vi "Teleop.vi"(10 "Match Info":T1={"Autonomous Elapsed Seconds"=0.0, "TeleOp Elapsed Seconds"=0.0, "Disabled Elapsed Seconds"=0.0, "Visited Autonomous"=FALSE, "Visited TeleOp"=FALSE, "Visited Disabled"=FALSE, "Autonomous Settings"={"Autonomous Style"=enum."Independent", "VI Refnum"=refnum}}, 11 "Call Context":T2) -> ()   [LabVIEW 2015]
doc: "This VI is called for each TeleOp packet received from the DS where the robot is not disabled. It is often used to read from the joysticks and update I/O or to update setpoints for timed control loops. It should complete and return within 20 milliseconds or it may miss DS packets."
uses:
  <vilib>/Rock Robotics/WPI/DriverStation/WPI_DriverStationDerivedRobotMode.ctl
  <vilib>/Rock Robotics/WPI/DriverStation/WPI_DriverStationMatch Info.ctl
  <vilib>/Rock Robotics/WPI/Solenoid/WPI_SolenoidValue.ctl
  <vilib>/Rock Robotics/WPI/Utilities/WPI_GetSetVariantRefNum.vi
  <vilib>/Rock Robotics/Network Tables/NT Write Boolean Array.vi
  <vilib>/Rock Robotics/Network Tables/NT Write Numeric Array.vi
  <vilib>/Rock Robotics/Network Tables/NT Read Boolean.vi
  <vilib>/Rock Robotics/Network Tables/NT Read Number.vi
  Robot Global Data.vi
  <vilib>/Rock Robotics/WPI/Solenoid/WPI_SolenoidSetEnum.vi
panel:
  in  "Delay (ms)":u32=5000
  in  "ArmFactor":dbl=1.0
  in  "y":dbl
  in  "WinchFactor":dbl=-1.0 format="%#_13g"
  in  "SquareInput?":bool
  in  "Rumble":sgl
  out "Sample Slider 0":dbl(slide) scale=0.0..5.0
  out "Sample Boolean 1":bool
  out "Sample Boolean 0":bool
  # "h"
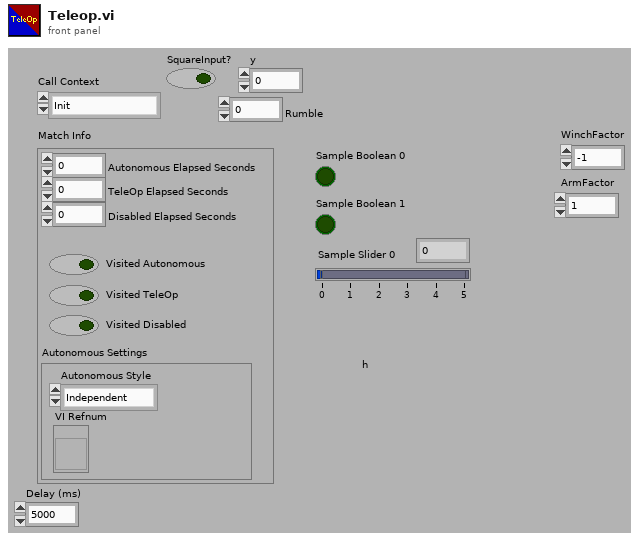
[diagram p1: front panel]
types:
  T1 = typedef "WPI_DriverStationMatch Info.ctl" = cluster{"Autonomous Elapsed Seconds":dbl, "TeleOp Elapsed Seconds":dbl, "Disabled Elapsed Seconds":dbl, "Visited Autonomous":bool, "Visited TeleOp":bool, "Visited Disabled":bool, "Autonomous Settings":cluster{"Autonomous Style":enum16{"Iterative", "Independent"}, "VI Refnum":refnum<vi>}}
  T2 = typedef "WPI_DriverStationDerivedRobotMode.ctl" = enum16{"Init", "Execute", "Stop"}
  T3 = cluster{"Distance (ft)":dbl, "Center":cluster{dbl, dbl}, "Normalized Rect":cluster{"Numeric":dbl, "Numeric 2":dbl, "Numeric 3":dbl, "Numeric 5":dbl}}[]
  T4 = cluster{"Detected Targets[0]":cluster{"Distance (ft)":dbl, "Center":cluster{dbl, dbl}, "Normalized Rect":cluster{"Numeric":dbl, "Numeric 2":dbl, "Numeric 3":dbl, "Numeric 5":dbl}}, "Detected Targets[1]":cluster{"Distance (ft)":dbl, "Center":cluster{dbl, dbl}, "Normalized Rect":cluster{"Numeric":dbl, "Numeric 2":dbl, "Numeric 3":dbl, "Numeric 5":dbl}}, "Detected Targets[2]":cluster{"Distance (ft)":dbl, "Center":cluster{dbl, dbl}, "Normalized Rect":cluster{"Numeric":dbl, "Numeric 2":dbl, "Numeric 3":dbl, "Numeric 5":dbl}}, "Detected Targets[3]":cluster{"Distance (ft)":dbl, "Center":cluster{dbl, dbl}, "Normalized Rect":cluster{"Numeric":dbl, "Numeric 2":dbl, "Numeric 3":dbl, "Numeric 5":dbl}}, "Detected Targets[4]":cluster{"Distance (ft)":dbl, "Center":cluster{dbl, dbl}, "Normalized Rect":cluster{"Numeric":dbl, "Numeric 2":dbl, "Numeric 3":dbl, "Numeric 5":dbl}}, "Detected Targets[5]":cluster{"Distance (ft)":dbl, "Center":cluster{dbl, dbl}, "Normalized Rect":cluster{"Numeric":dbl, "Numeric 2":dbl, "Numeric 3":dbl, "Numeric 5":dbl}}, "Detected Targets[6]":cluster{"Distance (ft)":dbl, "Center":cluster{dbl, dbl}, "Normalized Rect":cluster{"Numeric":dbl, "Numeric 2":dbl, "Numeric 3":dbl, "Numeric 5":dbl}}, "Detected Targets[7]":cluster{"Distance (ft)":dbl, "Center":cluster{dbl, dbl}, "Normalized Rect":cluster{"Numeric":dbl, "Numeric 2":dbl, "Numeric 3":dbl, "Numeric 5":dbl}}, "Detected Targets[8]":cluster{"Distance (ft)":dbl, "Center":cluster{dbl, dbl}, "Normalized Rect":cluster{"Numeric":dbl, "Numeric 2":dbl, "Numeric 3":dbl, "Numeric 5":dbl}}}
  T5 = typedef "WPI_JoystickDevRef.ctl" = cluster{"Device":T6}
  T6 = typedef "WPI_JoystickDeviceEnum.ctl" = enum16{"USB 0", "USB 1", "USB 2", "USB 3", "USB 4", "USB 5"}
  T7 = cluster{"Buttons[0]":bool, "Buttons[1]":bool, "Buttons[2]":bool, "Buttons[3]":bool, "Buttons[4]":bool, "Buttons[5]":bool, "Buttons[6]":bool, "Buttons[7]":bool, "Buttons[8]":bool, "Buttons[9]":bool}
  T8 = cluster{"Buttons[0]":bool, "Buttons[1]":bool, "Buttons[2]":bool, "Buttons[3]":bool, "Buttons[4]":bool, "Buttons[5]":bool, "Buttons[6]":bool, "Buttons[7]":bool, "Buttons[8]":bool}
  T9 = cluster{"Axes[0]":dbl, "Axes[1]":dbl, "Axes[2]":dbl, "Axes[3]":dbl, "Axes[4]":dbl, "Axes[5]":dbl, "Axes[6]":dbl, "Axes[7]":dbl, "Axes[8]":dbl}
  T10 = cluster{"TopLeft":bool, "TopCenter":bool, "TopRight":bool, "MiddleRight":bool, "MiddleLeft":bool, "MiddleCenter":bool, "BottomRight":bool, "BottomLeft":bool, "BottomCenter":bool, "Top":bool, "Middle":bool, "Bottom":bool, "Left":bool, "Center":bool, "Right":bool}
  T11 = typedef "WPI_SolenoidValue.ctl" = enum16{"Off", "On", "Forward", "Reverse"}
  T12 = typedef "WPI_SolenoidDevRef.ctl" = cluster{"DevStatus":errorcluster, "Pneumatics Control Module":u8, "Forward Solenoid Channel":T13, "Reverse Solenoid Channel":T13}
  T13 = typedef "WPI_SolenoidChannel.ctl" = enum8{"Solenoid 0", "Solenoid 1", "Solenoid 2", "Solenoid 3", "Solenoid 4", "Solenoid 5", "Solenoid 6", "Solenoid 7", "Invalid"}
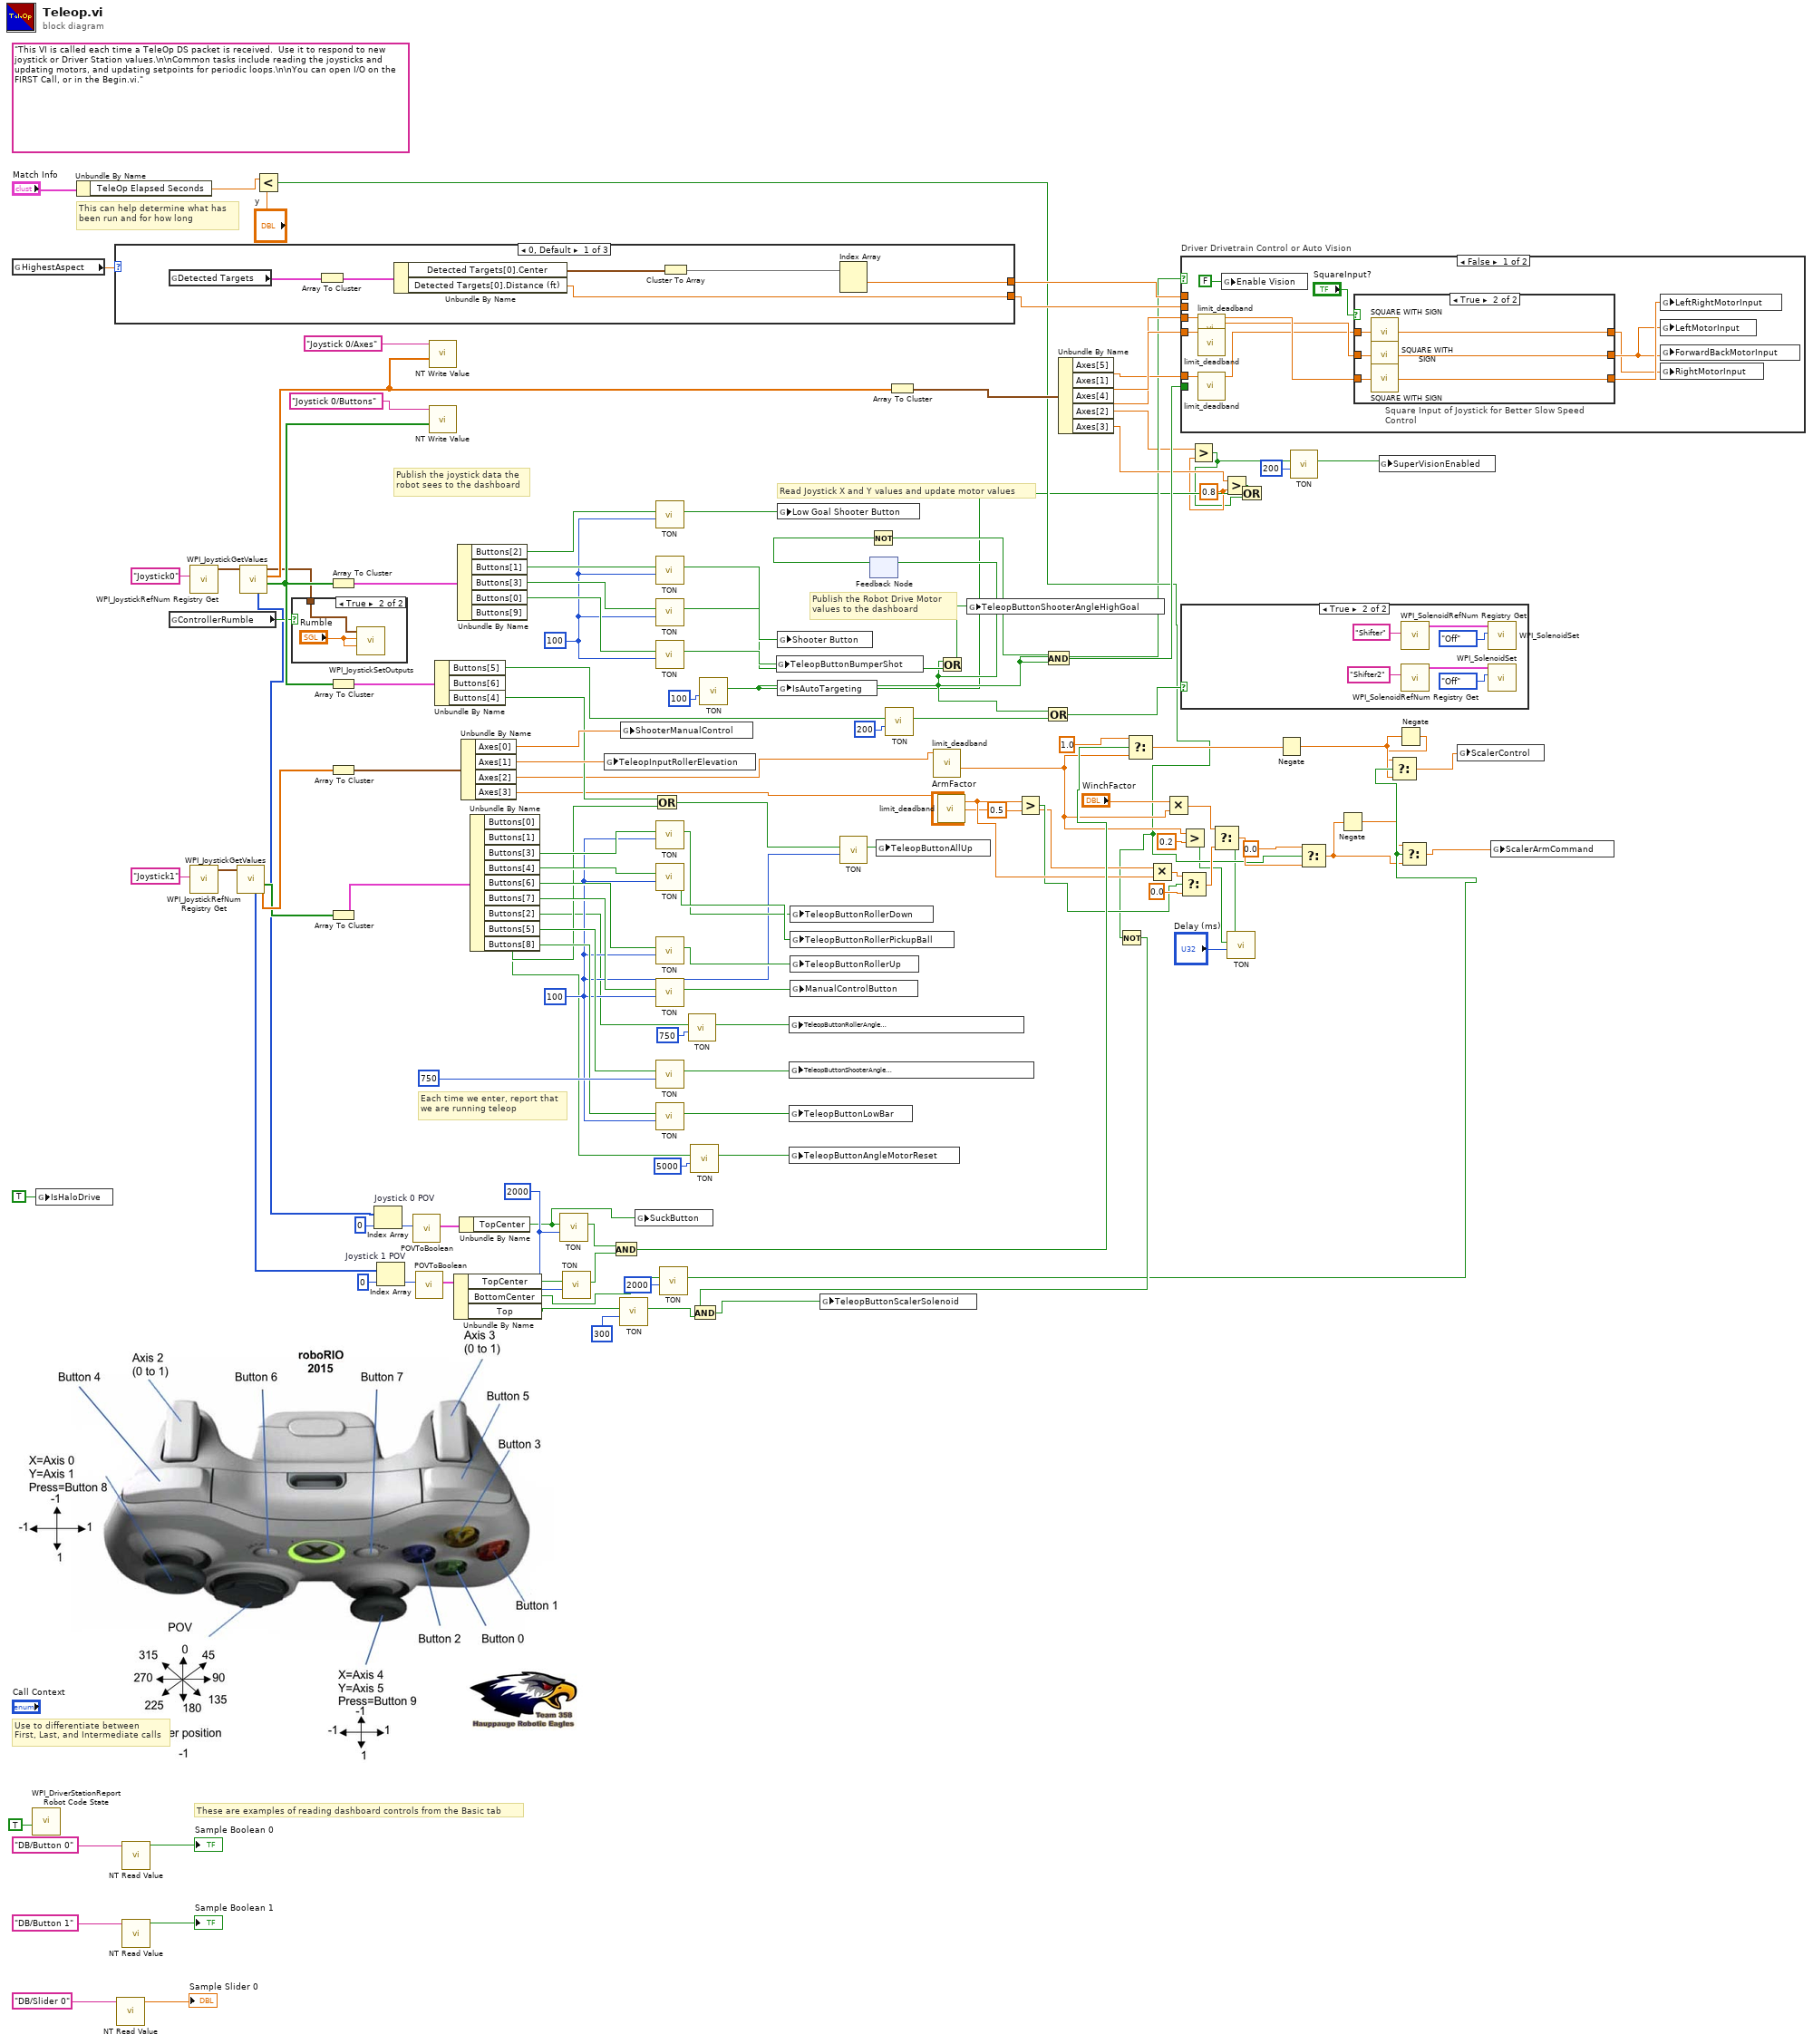
[diagram p0: block diagram]
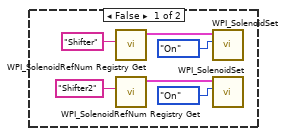
[diagram p3: hidden frame]
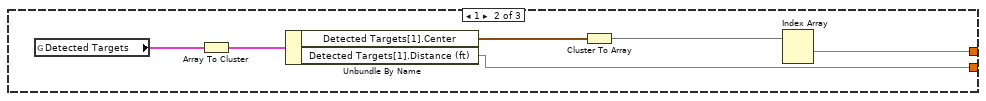
[diagram p4: hidden frame]
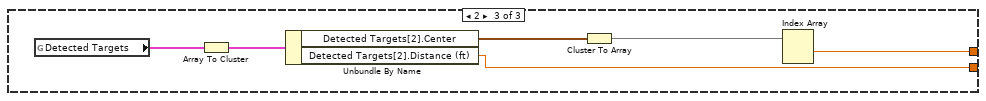
[diagram p5: hidden frame]
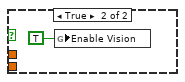
[diagram p7: hidden frame]
diagram:
  w4 = 0.8 ("y")
  w51 = u32 2000 ("Delay (ms)")
  w82 = u32 100 ("Delay (ms)")
  w75 = u32 100 ("Delay (ms)")
  (unwired) "This VI is called each time a TeleOp DS packet is received.  Use it to respond to new joystick or Driver Station values.\n\nCommon tasks include reading the joysticks and updating motors, and updating setpoints for periodic loops.\n\nYou can open I/O on the FIRST Call, or in the Begin.vi."
  # "These are examples of reading dashboard controls from the Basic tab"
  # "Publish the Robot Drive Motor\nvalues to the dashboard"
  # "Publish the joystick data the\nrobot sees to the dashboard"
  # "Each time we enter, report that\nwe are running teleop"
  # "Use to differentiate between\nFirst, Last, and Intermediate calls"
  # "This can help determine what has\nbeen run and for how long"
  # "Read Joystick X and Y values and update motor values"
  n1 = global read "Robot Global Data.vi" "HighestAspect"() -> (w120:dbl)
  n2 = call <vilib>:"WPI_DriverStationReport Robot Code State.vi"("TeleOp"=TRUE ("Autonomous")) -> ()  [unwired: 10 in, 1 out]
  n3 = global write "Robot Global Data.vi" "IsHaloDrive"(TRUE ("IsHaloDrive")) -> ()
  n4 = Unbundle By Name("Match Info") -> ("TeleOp Elapsed Seconds"=w34:dbl)
  n5 = case shown="0, Default" w120 {
    tunnel: [w138 w144 w150] -> w122
    tunnel: [w137 w143 w149] -> w121
    frame 0, Default {
      n6 = global read "Robot Global Data.vi" "Detected Targets"() -> (w139:T3)
      n7 = Array To Cluster(array=w139) -> (cluster=w142:T4)
      n8 = Unbundle By Name(w142) -> ("Detected Targets[0].Center"=w141:cluster{dbl, dbl}, "Detected Targets[0].Distance (ft)"=w137:dbl)
      n9 = Cluster To Array(cluster=w141) -> (array=w140:dbl[])
      n10 = Index Array(array=w140) -> (element #1=w138:dbl)  [unwired: 2 in, 1 out]
    }
    frame 1 {
      n11 = global read "Robot Global Data.vi" "Detected Targets"() -> (w145:T3)
      n12 = Array To Cluster(array=w145) -> (cluster=w148:T4)
      n13 = Unbundle By Name(w148) -> ("Detected Targets[1].Center"=w147:cluster{dbl, dbl}, "Detected Targets[1].Distance (ft)"=w143:dbl)
      n14 = Cluster To Array(cluster=w147) -> (array=w146:dbl[])
      n15 = Index Array(array=w146) -> (element #1=w144:dbl)  [unwired: 2 in, 1 out]
    }
    frame 2 {
      n16 = global read "Robot Global Data.vi" "Detected Targets"() -> (w151:T3)
      n17 = Array To Cluster(array=w151) -> (cluster=w154:T4)
      n18 = Unbundle By Name(w154) -> ("Detected Targets[2].Center"=w153:cluster{dbl, dbl}, "Detected Targets[2].Distance (ft)"=w149:dbl)
      n19 = Cluster To Array(cluster=w153) -> (array=w152:dbl[])
      n20 = Index Array(array=w152) -> (element #1=w150:dbl)  [unwired: 2 in, 1 out]
    }
  }
  n21 = call-poly <vilib>:"NT Read Value.vi"("Name"="DB/Slider 0" ("refnum name")) -> ("Numeric"=→"Sample Slider 0":dbl)  [unwired: 9 in, 1 out]
  n22 = call-poly <vilib>:"NT Read Value.vi"("Name"="DB/Button 0" ("refnum name")) -> ("Boolean"=→"Sample Boolean 0":bool)  [unwired: 9 in, 1 out]
  n23 = call-poly <vilib>:"NT Read Value.vi"("Name"="DB/Button 1" ("refnum name")) -> ("Boolean"=→"Sample Boolean 1":bool)  [unwired: 9 in, 1 out]
  n24 = global read "Robot Global Data.vi" "ControllerRumble"() -> (w62:bool)
  n25 = call <vilib>:"WPI_JoystickRefNum Registry Get.vi"("refnum name"="Joystick0") -> ("JoystickDevRef"=w134:T5)  [unwired: 1 in, 9 out]
  n26 = call <vilib>:"WPI_JoystickRefNum Registry Get.vi"("refnum name"="Joystick1") -> ("JoystickDevRef"=w105:T5)  [unwired: 1 in, 9 out]
  n27 = call <vilib>:"WPI_JoystickGetValues.vi"("JoystickDevRef"=w105) -> ("Buttons"=w102:bool[], "Axes"=w104:dbl[], "POVs"=w53:i16[])  [unwired: 6 in, 2 out]
  n28 = call <vilib>:"WPI_JoystickGetValues.vi"("JoystickDevRef"=w134) -> ("Buttons"=w110:bool[], "Axes"=w131:dbl[], "JoystickDevRef"=w61:T5, "POVs"=w57:i16[])  [unwired: 6 in, 1 out]
  n29 = Less?(x=w34, y="y") -> (x < y?=w24:bool)
  n30 = case shown="True" w62 {
    tunnel: w61 -> [_ w155]
    frame False {
    }
    frame True {
      n31 = call <vilib>:"WPI_JoystickSetOutputs.vi"("Right Rumble"="Rumble", "Left Rumble"="Rumble", "JoystickDevRef"=w155) -> ()  [unwired: 7 in, 2 out]
    }
  }
  n32 = Array To Cluster(array=w110) -> (cluster=w109:T7)
  n33 = Array To Cluster(array=w110) -> (cluster=w123:T8)
  n34 = Array To Cluster(array=w104) -> (cluster=w103:T9)
  n35 = Array To Cluster(array=w102) -> (cluster=w101:T8)
  n36 = Index Array "Joystick 0 POV"(array=w57, index=0) -> (element=w59:i16)
  n37 = Index Array "Joystick 1 POV"(array=w53, index=0) -> (element=w55:i16)
  n38 = call "POVToBoolean.vi"("Input"=w59) -> ("Output"=w58:T10)  [unwired: 10 in]
  n39 = call "POVToBoolean.vi"("Input"=w55) -> ("Output"=w54:T10)  [unwired: 10 in]
  n40 = call-poly <vilib>:"NT Write Value.vi"("Numeric Array"=w131, "Name"="Joystick 0/Axes") -> ()  [unwired: 9 in, 1 out]
  n41 = call-poly <vilib>:"NT Write Value.vi"("Boolean Array"=w110, "Name"="Joystick 0/Buttons") -> ()  [unwired: 9 in, 1 out]
  n42 = Unbundle By Name(w123) -> ("Buttons[5]"=w118:bool, "Buttons[4]"=w76:bool)  [unwired: 1 out]
  n43 = Unbundle By Name(w54) -> ("TopCenter"=w52:bool, "BottomCenter"=w21:bool, "Top"=w36:bool)
  n44 = Unbundle By Name(w109) -> ("Buttons[2]"=w77:bool, "Buttons[1]"=w108:bool, "Buttons[3]"=w107:bool, "Buttons[0]"=w83:bool)  [unwired: 1 out]
  n45 = Unbundle By Name(w58) -> ("TopCenter"=w7:bool)
  n46 = Unbundle By Name(w103) -> ("Axes[0]"=w89:dbl, "Axes[1]"=w88:dbl, "Axes[2]"=w64:dbl, "Axes[3]"=w63:dbl)
  n47 = Unbundle By Name(w101) -> ("Buttons[0]"=w97:bool, "Buttons[1]"=w96:bool, "Buttons[3]"=w95:bool, "Buttons[4]"=w85:bool, "Buttons[6]"=w73:bool, "Buttons[7]"=w90:bool, "Buttons[2]"=w86:bool, "Buttons[5]"=w80:bool, "Buttons[8]"=w71:bool)
  n48 = call "TON.vi"("Delay (ms)"=w51, "Input"=w7) -> ("Output"=w50:bool)  [unwired: 9 in]
  n49 = call "TON.vi"("Delay (ms)"=w51, "Input"=w52) -> ("Output"=w49:bool)  [unwired: 9 in]
  n50 = global write "Robot Global Data.vi" "TeleopInputRollerElevation"(w88) -> ()
  n51 = And(x=w50, y=w49) -> (x .and. y?=w48:bool)
  n52 = call "TON.vi"("Delay (ms)"=u32 300, "Input"=w36) -> ("Output"=w33:bool)  [unwired: 9 in]
  n53 = global write "Robot Global Data.vi" "ShooterManualControl"(w89) -> ()
  n54 = global write "Robot Global Data.vi" "SuckButton"(w7) -> ()
  n55 = Or(x=w76, y=w80) -> (x .or. y?=w79:bool)
  n56 = call "TON.vi"("Delay (ms)"=w75, "Input"=w77) -> ("Output"=w113:bool)  [unwired: 9 in]
  n57 = call "TON.vi"("Delay (ms)"=w75, "Input"=w108) -> ("Output"=w35:bool)  [unwired: 9 in]
  n58 = call "TON.vi"("Delay (ms)"=w75, "Input"=w107) -> ("Output"=w112:bool)  [unwired: 9 in]
  n59 = call "TON.vi"("Delay (ms)"=w75, "Input"=w83) -> ("Output"=w111:bool)  [unwired: 9 in]
  n60 = call "TON.vi"("Delay (ms)"=w82, "Input"=w97) -> ("Output"=w98:bool)  [unwired: 9 in]
  n61 = call "TON.vi"("Delay (ms)"=w82, "Input"=w96) -> ("Output"=w100:bool)  [unwired: 9 in]
  n62 = call "TON.vi"("Delay (ms)"=w82, "Input"=w95) -> ("Output"=w99:bool)  [unwired: 9 in]
  n63 = call "TON.vi"("Delay (ms)"=w82, "Input"=w85) -> ("Output"=w84:bool)  [unwired: 9 in]
  n64 = call "TON.vi"("Delay (ms)"=u32 750, "Input"=w90) -> ("Output"=w92:bool)  [unwired: 9 in]
  n65 = call "TON.vi"("Delay (ms)"=w82, "Input"=w86) -> ("Output"=w87:bool)  [unwired: 9 in]
  n66 = call "TON.vi"("Delay (ms)"=u32 2000, "Input"=w21) -> ("Output"=w19:bool)  [unwired: 9 in]
  n67 = call "TON.vi"("Delay (ms)"=u32 750, "Input"=w73) -> ("Output"=w94:bool)  [unwired: 9 in]
  n68 = call "TON.vi"("Delay (ms)"=u32 5000, "Input"=w71) -> ("Output"=w70:bool)  [unwired: 9 in]
  n69 = global write "Robot Global Data.vi" "TeleopButtonBumperShot"(w111) -> ()
  n70 = global write "Robot Global Data.vi" "Low Goal Shooter Button"(w113) -> ()
  n71 = global write "Robot Global Data.vi" "Shooter Button"(w112) -> ()
  n72 = global write "Robot Global Data.vi" "TeleopButtonRollerAngle\nEmergencyManual"(w94) -> ()
  n73 = global write "Robot Global Data.vi" "TeleopButtonShooterAngle\nEmergencyManual"(w92) -> ()
  n74 = global write "Robot Global Data.vi" "TeleopButtonLowBar"(w87) -> ()
  n75 = global write "Robot Global Data.vi" "TeleopButtonAngleMotorReset"(w70) -> ()
  n76 = global write "Robot Global Data.vi" "TeleopButtonRollerDown"(w98) -> ()
  n77 = global write "Robot Global Data.vi" "TeleopButtonRollerPickupBall"(w100) -> ()
  n78 = global write "Robot Global Data.vi" "TeleopButtonRollerUp"(w99) -> ()
  n79 = global write "Robot Global Data.vi" "ManualControlButton"(w84) -> ()
  n80 = call "TON.vi"("Delay (ms)"=w82, "Input"=w79) -> ("Output"=w81:bool)  [unwired: 9 in]
  n81 = feedback #1() -> (w67:bool)  [unwired: 1 in]
  n82 = Not(x=w67) -> (.not. x?=w69:bool)
  n83 = global write "Robot Global Data.vi" "TeleopButtonAllUp"(w81) -> ()
  n84 = call "TON.vi"("Delay (ms)"=u32 200, "Input"=w118) -> ("Output"=w66:bool)  [unwired: 9 in]
  n85 = Array To Cluster(array=w131) -> (cluster=w117:T9)
  n86 = call "limit_deadband.vi"("Val"=w64) -> ("Val Out"=w39:dbl)  [unwired: 10 in]
  n87 = call "limit_deadband.vi"("Val"=w63) -> ("Val Out"=w43:dbl)  [unwired: 10 in]
  n88 = Greater?(x=w43, y=0.5) -> (0:w27:bool)
  n89 = Unbundle By Name(w117) -> ("Axes[5]"=w114:dbl, "Axes[1]"=w116:dbl, "Axes[4]"=w115:dbl, "Axes[2]"=w5:dbl, "Axes[3]"=w14:dbl)
  n90 = Not(x=w24) -> (.not. x?=w32:bool)
  n91 = And(x=w32, y=w33) -> (x .and. y?=w31:bool)
  n92 = global write "Robot Global Data.vi" "TeleopButtonScalerSolenoid"(w31) -> ()
  n93 = Select(t=1.0, s=w48, f=w39) -> (s? t:f=w30:dbl)
  n94 = Multiply(x="ArmFactor", y=w43) -> (x*y=w44:dbl)
  n95 = Multiply(x="WinchFactor", y=w39) -> (x*y=w38:dbl)
  n96 = Select(t=w44, s=w27, f=0.0) -> (s? t:f=w41:dbl)
  n97 = Greater?(x=w39, y=0.2) -> (0:w10:bool)
  n98 = Greater?(x=w5, y=w4) -> (0:w3:bool)
  n99 = Greater?(x=w14, y=w4) -> (0:w13:bool)
  n100 = call "TON.vi"("Delay (ms)"="Delay (ms)", "Input"=w10) -> ("Output"=w9:bool)  [unwired: 9 in]
  n101 = Select(t=w38, s=w9, f=w41) -> (s? t:f=w28:dbl)
  n102 = Or(x=w13, y=w3) -> (x .or. y?=w6:bool)
  n103 = call "TON.vi"("Delay (ms)"=u32 100, "Input"=w6) -> ("Output"=w11:bool)  [unwired: 9 in]
  n104 = global write "Robot Global Data.vi" "IsAutoTargeting"(w11) -> ()
  n105 = feedback-in #1(w11) -> ()
  n106 = Or(x=w11, y=w35) -> (x .or. y?=w12:bool)
  n107 = global write "Robot Global Data.vi" "TeleopButtonShooterAngleHighGoal"(w12) -> ()
  n108 = Or(x=w11, y=w66) -> (x .or. y?=w65:bool)
  n109 = And(x=w69, y=w11) -> (x .and. y?=w68:bool)
  n110 = case "Driver Drivetrain Control or Auto Vision" shown="False" w11 {
    tunnel: w122 -> [_ _]
    tunnel: w121 -> [_ _]
    tunnel: w116 -> [w165 _]
    tunnel: w115 -> [w164 _]
    tunnel: w114 -> [w166 _]
    tunnel: w68 -> [_ _]
    frame False {
      n111 = call "limit_deadband.vi"("Val"=w164) -> ("Val Out"=w162:dbl)  [unwired: 10 in]
      n112 = call "limit_deadband.vi"("Val"=w165) -> ("Val Out"=w161:dbl)  [unwired: 10 in]
      n113 = call "limit_deadband.vi"("Val"=w166) -> ("Val Out"=w160:dbl)  [unwired: 10 in]
      n114 = global write "Robot Global Data.vi" "Enable Vision"(FALSE ("Enable Vision")) -> ()
      n115 = case "Square Input of Joystick for Better Slow Speed Control" shown="True" "SquareInput?" {
        tunnel: w162 -> [w170 w176]
        tunnel: w161 -> [w169 w175]
        tunnel: w160 -> [w168 w174]
        tunnel: [w170 w173] -> w159
        tunnel: [w169 w172] -> w158
        tunnel: [w168 w171] -> w157
        frame False {
        }
        frame True {
          n116 = call "SQUARE WITH SIGN.vi"("Input"=w174) -> ("Output"=w171:dbl)
          n117 = call "SQUARE WITH SIGN.vi"("Input"=w175) -> ("Output"=w172:dbl)
          n118 = call "SQUARE WITH SIGN.vi"("Input"=w176) -> ("Output"=w173:dbl)
        }
      }
      n119 = global write "Robot Global Data.vi" "LeftRightMotorInput"(w159) -> ()
      n120 = global write "Robot Global Data.vi" "LeftMotorInput"(w158) -> ()
      n121 = global write "Robot Global Data.vi" "ForwardBackMotorInput"(w158) -> ()
      n122 = global write "Robot Global Data.vi" "RightMotorInput"(w157) -> ()
    }
    frame True {
      n123 = global write "Robot Global Data.vi" "Enable Vision"(TRUE ("Enable Vision")) -> ()
    }
  }
  n124 = case shown="True" w65 {
    frame False {
      n125 = call <vilib>:"WPI_SolenoidRefNum Registry Get.vi"("refnum name"="Shifter") -> ("SolenoidDevRef"=w181:T12)  [unwired: 9 in, 1 out]
      n126 = call <vilib>:"WPI_SolenoidRefNum Registry Get.vi"("refnum name"="Shifter2") -> ("SolenoidDevRef"=w178:T12)  [unwired: 9 in, 1 out]
      n127 = call-poly <vilib>:"WPI_SolenoidSet.vi"("Value"=WPI_SolenoidValue."On", "SolenoidDevRef"=w181) -> ()  [unwired: 8 in, 2 out]
      n128 = call-poly <vilib>:"WPI_SolenoidSet.vi"("Value"=WPI_SolenoidValue."On", "SolenoidDevRef"=w178) -> ()  [unwired: 8 in, 2 out]
    }
    frame True {
      n129 = call <vilib>:"WPI_SolenoidRefNum Registry Get.vi"("refnum name"="Shifter") -> ("SolenoidDevRef"=w187:T12)  [unwired: 9 in, 1 out]
      n130 = call <vilib>:"WPI_SolenoidRefNum Registry Get.vi"("refnum name"="Shifter2") -> ("SolenoidDevRef"=w184:T12)  [unwired: 9 in, 1 out]
      n131 = call-poly <vilib>:"WPI_SolenoidSet.vi"("Value"=WPI_SolenoidValue."Off", "SolenoidDevRef"=w187) -> ()  [unwired: 8 in, 2 out]
      n132 = call-poly <vilib>:"WPI_SolenoidSet.vi"("Value"=WPI_SolenoidValue."Off", "SolenoidDevRef"=w184) -> ()  [unwired: 8 in, 2 out]
    }
  }
  n133 = Negate(x=w30) -> (-x=w18:dbl)
  n134 = call "TON.vi"("Delay (ms)"=u32 200, "Input"=w3) -> ("Output"=w2:bool)  [unwired: 9 in]
  n135 = Select(t=0.0, s=w24, f=w28) -> (s? t:f=w16:dbl)
  n136 = Negate(x=w16) -> (-x=w15:dbl)
  n137 = global write "Robot Global Data.vi" "SuperVisionEnabled"(w2) -> ()
  n138 = Negate(x=w18) -> (-x=w17:dbl)
  n139 = Select(t=w17, s=w19, f=w18) -> (s? t:f=w23:dbl)
  n140 = Select(t=w15, s=w19, f=w16) -> (s? t:f=w22:dbl)
  n141 = global write "Robot Global Data.vi" "ScalerControl"(w23) -> ()
  n142 = global write "Robot Global Data.vi" "ScalerArmCommand"(w22) -> ()
